vi "Read AO task.vi"(8 "error in (no error)":errorcluster, 11 "DAQmx Synthesizer in":refnum<class "DAQmx Synthesizer.lvclass">) -> (0 "error out":errorcluster, 2 "AO task":refnum<k21>, 3 "DAQmx Synthesizer out":refnum<class "DAQmx Synthesizer.lvclass">)   [LabVIEW 2021, in "DAQmx Synthesizer.lvclass"]
uses:
  DAQmx Synthesizer.lvclass
  DAQmx Synthesizer.lvclass/DAQmx Synthesizer.ctl
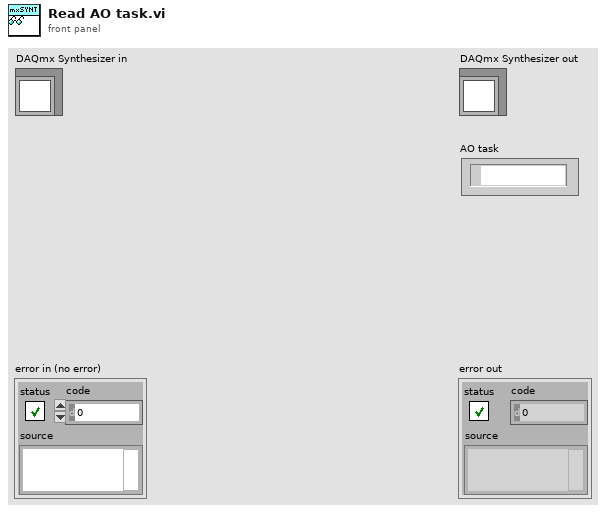
[diagram p1: front panel]
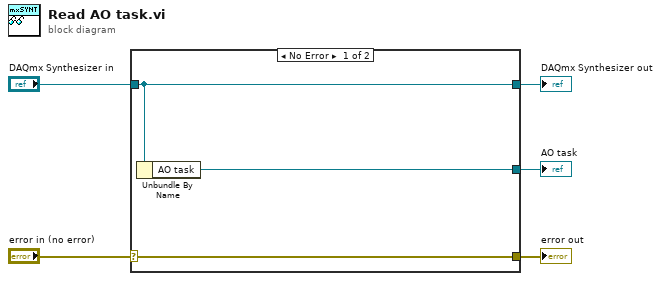
[diagram p0: block diagram]
diagram:
  n1 = case shown="No Error" "error in (no error)" {
    selector: "error in (no error)" -> [w8 w9]
    tunnel: [w8 w9] -> w4
    tunnel: [w7 w10] -> w2
    tunnel: "DAQmx Synthesizer in" -> [w7 w10]
    tunnel: [w6 _] -> w1
    frame No Error {
      n2 = Unbundle By Name(w7) -> ("AO task"=w6:refnum<k21>)
    }
    frame Error {
    }
  }
  "error out" <- w4
  "DAQmx Synthesizer out" <- w2
  "AO task" <- w1
